vi "GetFrame.vi"(9 "timeoutMS":u32, 10 "handle":i64, 11 "error in (no error)":errorcluster) -> (0 "frameHandle":i64, 1 "pData":u8[](array[numeric]), 2 "pLbFrame out":T1, 3 "error out":errorcluster, 4 "return type":i32)   [LabVIEW 2016]
uses:
  MVSDKmd.dll
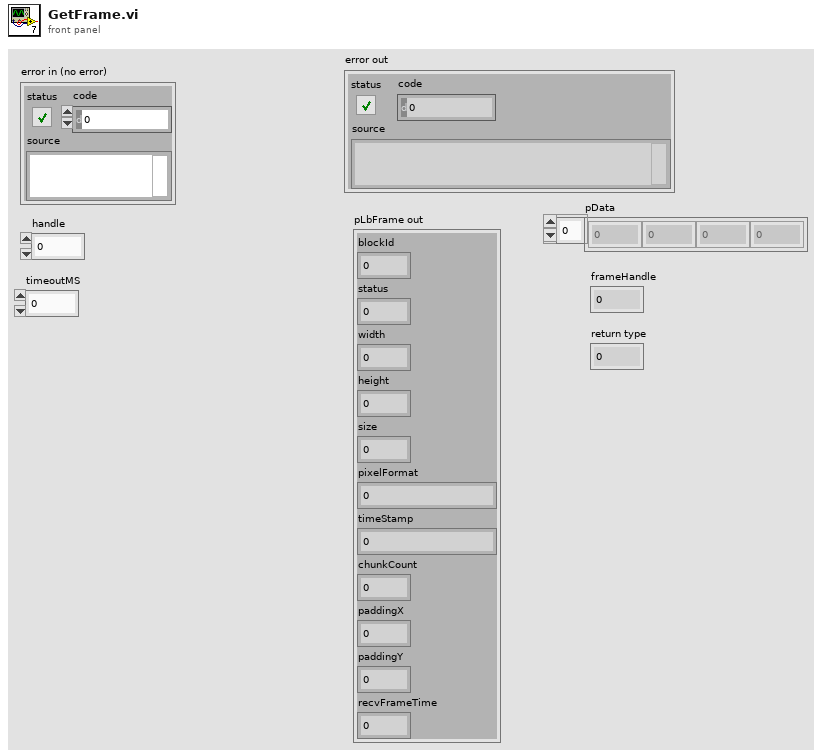
[diagram p1: front panel]
types:
  T1 = cluster{"blockId":u64, "status":u32, "width":u32, "height":u32, "size":u32, "pixelFormat":i32, "timeStamp":u64, "chunkCount":u32, "paddingX":u32, "paddingY":u32, "recvFrameTime":u32}
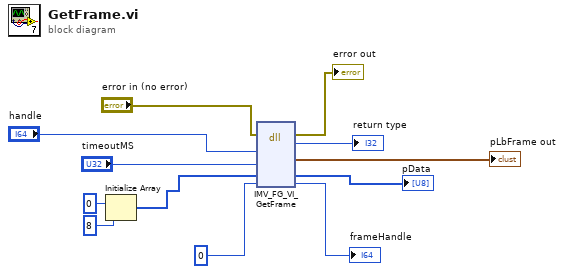
[diagram p0: block diagram]
diagram:
  n1 = Initialize Array(u8 0 ("element"), 8 ("dimension size")) -> (w2:u8[])
  n2 = dll-call lib="MVSDKmd.dll" fn="IMV_FG_VI_GetFrame"(error in="error in (no error)", "handle"="handle", "timeoutMS"="timeoutMS", "pData"=w2, "frameHandle"=i64 0) -> (error out=→"error out":errorcluster, "return type"=→"return type":i32, "pLbFrame out"=→"pLbFrame out":T1, "pData"=→"pData":u8[], "frameHandle"=→"frameHandle":i64)  [unwired: 5 in, 1 out]
